vi "N6701A_SetPSEnable.vi"(8 "error in (no error)":errorcluster, 9 "Enable Output (False)":bool, 10 "Channel Name (1)":string="2", 11 "VISA resource name":refnum<visa-resource-name>="PowerSupply2") -> (0 "error out":errorcluster)   [LabVIEW 2015]
uses:
  <instrlib>/Agilent N6700 Series/Agilent N6700 Series.lvlib
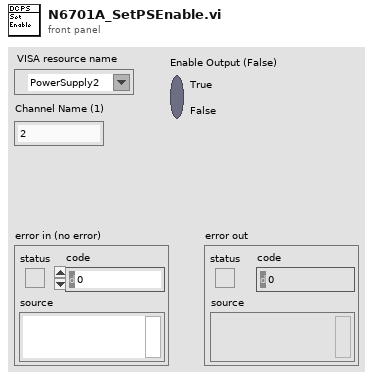
[diagram p1: front panel]
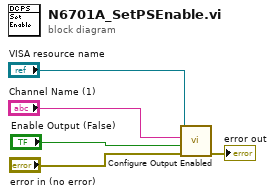
[diagram p0: block diagram]
diagram:
  n1 = call <instrlib>:"Configure Output Enabled.vi"("error in (no error)"="error in (no error)", "Enable Output (False)"="Enable Output (False)", "Channel Name (1)"="Channel Name (1)", "VISA resource name"="VISA resource name") -> ("error out"=→"error out":errorcluster)  [unwired: 6 in, 1 out]
